vi "Create Mask.vi"(8 "Combine Masks? (F)":bool, 9 "1-Bit Mask Value (T)":bool=TRUE, 10 "Mask Color (Black)":u32(colorbox), 11 "image data":T1) -> (3 "image data":T1)   [LabVIEW 2017]
doc: "Applies a mask to an image and returns the mask information in the <B>mask</B> element of <B>image data</B>. This VI is useful if you want to make a certain color in an image transparent before writing the image to a 2D picture control."
uses:
  imagedata.ctl
panel:
  in  "Case Constant\n(See Context Help)":bool=TRUE
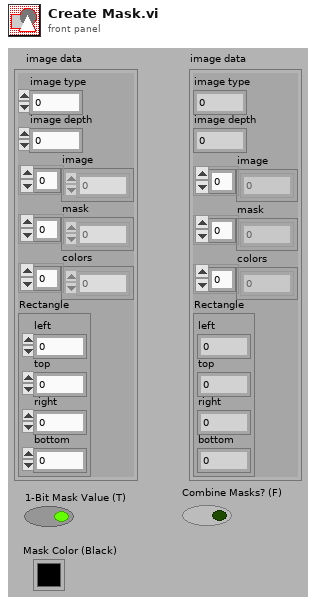
[diagram p1: front panel]
types:
  T1 = typedef "imagedata.ctl" = cluster{"image type":i32, "image depth":i32, "image":u8[], "mask":u8[], "colors":u32[], "Rectangle":cluster{"left":i16, "top":i16, "right":i16, "bottom":i16}}
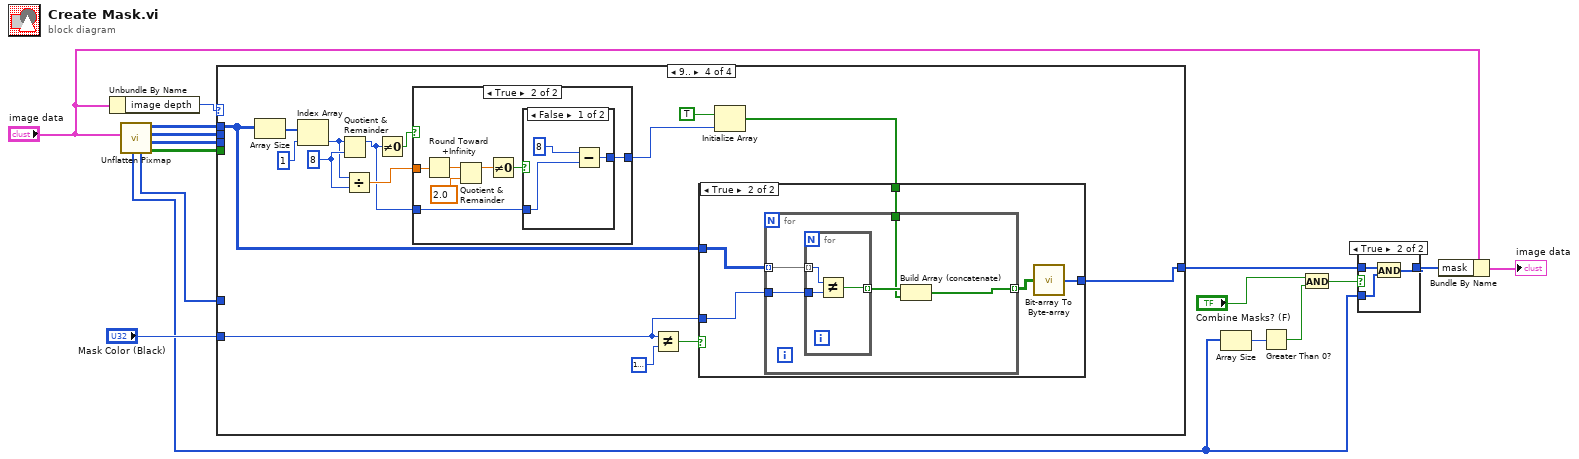
[diagram p0: block diagram]
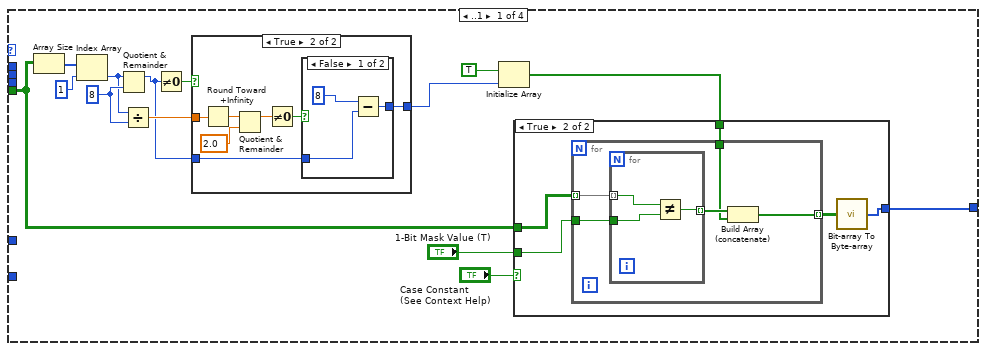
[diagram p3: hidden frame]
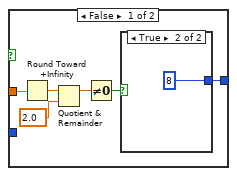
[diagram p4: hidden frame]
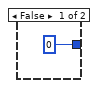
[diagram p5: hidden frame]
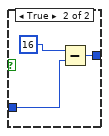
[diagram p6: hidden frame]
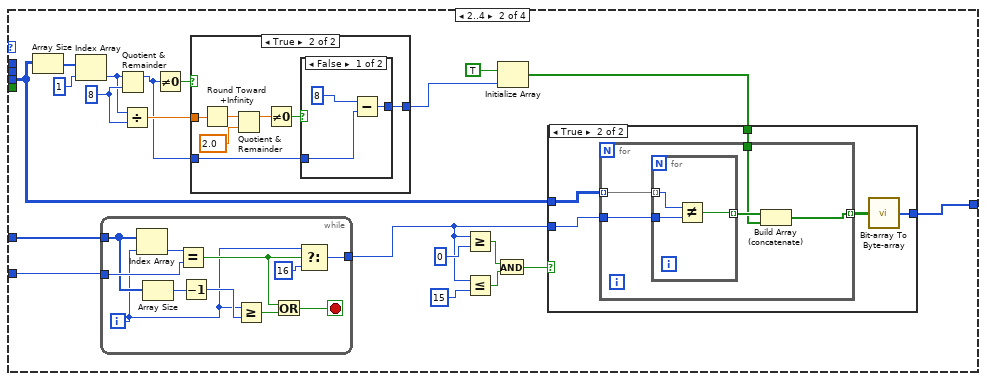
[diagram p8: hidden frame]
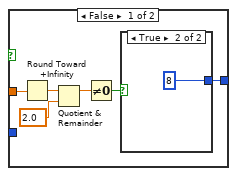
[diagram p9: hidden frame]
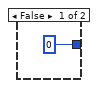
[diagram p10: hidden frame]
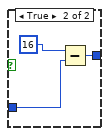
[diagram p11: hidden frame]
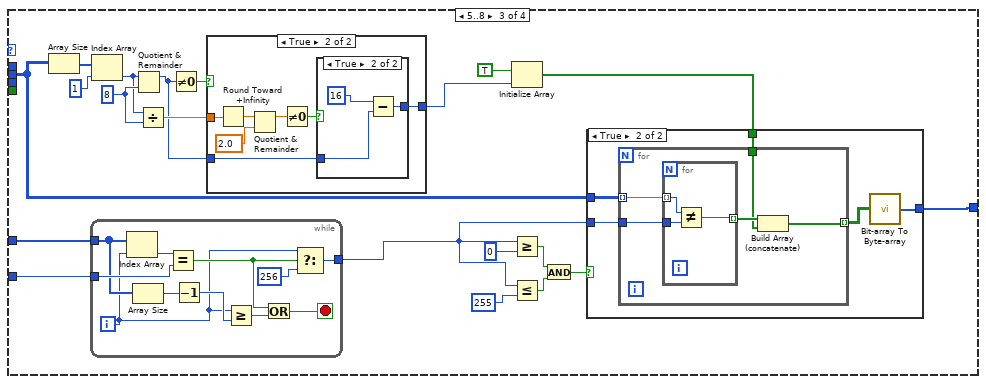
[diagram p13: hidden frame]
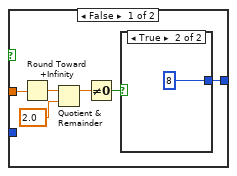
[diagram p14: hidden frame]
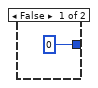
[diagram p15: hidden frame]
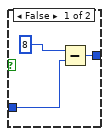
[diagram p16: hidden frame]
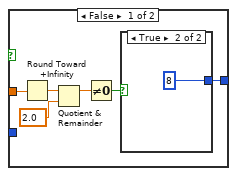
[diagram p18: hidden frame]
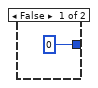
[diagram p19: hidden frame]
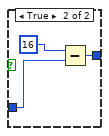
[diagram p20: hidden frame]
diagram:
  n1 = Unbundle By Name("image data") -> ("image depth"=w1:i32)
  n2 = call "Unflatten Pixmap.vi"("image data"="image data") -> ("1-bit pixmap"=w13:bool[][], "4-bit pixmap"=w14:u8[][], "8-bit pixmap"=w15:u8[][], "24-bit pixmap"=w16:u32[][], "colors"=w3:u32[], "mask"=w4:u8[])  [unwired: 4 in, 1 out]
  n3 = case shown="9.." w1 {
    tunnel: w15 -> [_ _ w140 _]
    tunnel: w14 -> [_ w77 _ _]
    tunnel: w13 -> [w24 _ _ _]
    tunnel: w16 -> [_ _ _ w198]
    tunnel: [w20 w71 w136 w200] -> w7
    tunnel: w3 -> [_ w70 w135 _]
    tunnel: "Mask Color (Black)" -> [_ w69 w134 w199]
    frame ..1 {
      w26 = 8 ("y")
      n4 = Array Size(array=w24) -> (size(s)=w28:i32[])
      n5 = Index Array(array=w28, index=1) -> (element=w22:i32)
      n6 = Quotient & Remainder(x=w22, y=w26) -> (x-y*floor(x/y)=w21:i32)  [unwired: 1 out]
      n7 = Divide(x=w22, y=w26) -> (x/y=w25:dbl)
      n8 = Not Equal To 0?(x=w21) -> (x != 0?=w27:bool)
      n9 = case shown="True" w27 {
        tunnel: w25 -> [w32 w45]
        tunnel: w21 -> [_ w40]
        tunnel: [w31 w39] -> w18
        frame False {
          n10 = Round Toward +Infinity(x=w32) -> (ceil(x): smallest int >= x=w33:dbl)
          n11 = Quotient & Remainder(x=w33, y=2.0) -> (x-y*floor(x/y)=w36:dbl)  [unwired: 1 out]
          n12 = Not Equal To 0?(x=w36) -> (x != 0?=w35:bool)
          n13 = case shown="True" w35 {
            tunnel: [0 8] -> w31
            frame False {
            }
            frame True {
            }
          }
        }
        frame True {
          n14 = Round Toward +Infinity(x=w45) -> (ceil(x): smallest int >= x=w44:dbl)
          n15 = Quotient & Remainder(x=w44, y=2.0) -> (x-y*floor(x/y)=w41:dbl)  [unwired: 1 out]
          n16 = Not Equal To 0?(x=w41) -> (x != 0?=w42:bool)
          n17 = case shown="False" w42 {
            tunnel: w40 -> [w46 w49]
            tunnel: [w47 w50] -> w39
            frame False {
              n18 = Subtract(x=8, y=w46) -> (x-y=w47:i32)
            }
            frame True {
              n19 = Subtract(x=16, y=w49) -> (x-y=w50:i32)
            }
          }
        }
      }
      n20 = Initialize Array(TRUE, w18) -> (w17:bool[])
      n21 = case shown="True" "Case Constant\n(See Context Help)" {
        tunnel: w24 -> [_ w56]
        tunnel: [_ w52] -> w20
        tunnel: "1-Bit Mask Value (T)" -> [_ w55]
        tunnel: w17 -> [_ w54]
        frame False {
        }
        frame True {
          n22 = for {
            tunnel: w56 -> [w61] mode=indexing
            tunnel: [w57] -> w53 mode=indexing
            tunnel: w55 -> [w60]
            tunnel: w54 -> [w58]
            n23 = for {
              tunnel: w61 -> [w62] mode=indexing
              tunnel: [w63] -> w59 mode=indexing
              tunnel: w60 -> [w64]
              n24 = Not Equal?(x=w62, y=w64) -> (x != y?=w63:bool)
            }
            n25 = Build Array (concatenate)(w59, w58) -> (w57:bool[])
          }
          n26 = call "Bit-array To Byte-array.vi"("bit array"=w53) -> ("byte array"=w52:u8[])
        }
      }
    }
    frame 2..4 {
      w79 = 8 ("y")
      n27 = Array Size(array=w77) -> (size(s)=w81:i32[])
      n28 = Index Array(array=w81, index=1) -> (element=w73:i32)
      n29 = while {
        tunnel: w70 -> [w93]
        tunnel: w69 -> [w94]
        tunnel: [w85] -> w68
        i -> [w87]
        stop <- w92 stop-if-true
        n30 = Index Array(array=w93, index=w87) -> (element=w95:u32)
        n31 = Array Size(array=w93) -> (size(s)=w90:i32)
        n32 = Equal?(x=w95, y=w94) -> (x = y?=w89:bool)
        n33 = Decrement(x=w90) -> (x-1=w88:i32)
        n34 = Greater Or Equal?(x=w87, y=w88) -> (x >= y?=w91:bool)
        n35 = Or(x=w89, y=w91) -> (x .or. y?=w92:bool)
        n36 = Select(t=w87, s=w89, f=16) -> (s? t:f=w85:i32)
      }
      n37 = Quotient & Remainder(x=w73, y=w79) -> (x-y*floor(x/y)=w72:i32)  [unwired: 1 out]
      n38 = Divide(x=w73, y=w79) -> (x/y=w78:dbl)
      n39 = Not Equal To 0?(x=w72) -> (x != 0?=w80:bool)
      n40 = case shown="True" w80 {
        tunnel: w78 -> [w97 w110]
        tunnel: w72 -> [_ w105]
        tunnel: [w96 w104] -> w66
        frame False {
          n41 = Round Toward +Infinity(x=w97) -> (ceil(x): smallest int >= x=w98:dbl)
          n42 = Quotient & Remainder(x=w98, y=2.0) -> (x-y*floor(x/y)=w101:dbl)  [unwired: 1 out]
          n43 = Not Equal To 0?(x=w101) -> (x != 0?=w100:bool)
          n44 = case shown="True" w100 {
            tunnel: [0 8] -> w96
            frame False {
            }
            frame True {
            }
          }
        }
        frame True {
          n45 = Round Toward +Infinity(x=w110) -> (ceil(x): smallest int >= x=w109:dbl)
          n46 = Quotient & Remainder(x=w109, y=2.0) -> (x-y*floor(x/y)=w106:dbl)  [unwired: 1 out]
          n47 = Not Equal To 0?(x=w106) -> (x != 0?=w107:bool)
          n48 = case shown="False" w107 {
            tunnel: w105 -> [w111 w114]
            tunnel: [w112 w115] -> w104
            frame False {
              n49 = Subtract(x=8, y=w111) -> (x-y=w112:i32)
            }
            frame True {
              n50 = Subtract(x=16, y=w114) -> (x-y=w115:i32)
            }
          }
        }
      }
      n51 = Greater Or Equal?(x=w68, y=u8 0) -> (x >= y?=w76:bool)
      n52 = Less Or Equal?(x=w68, y=u8 15) -> (x <= y?=w75:bool)
      n53 = And(x=w76, y=w75) -> (x .and. y?=w84:bool)
      n54 = Initialize Array(TRUE, w66) -> (w65:bool[])
      n55 = case shown="True" w84 {
        tunnel: w77 -> [_ w121]
        tunnel: w68 -> [_ w120]
        tunnel: w65 -> [_ w119]
        tunnel: [_ w117] -> w71
        frame False {
          (unwired) i16 0
          (unwired) i16 0
        }
        frame True {
          n56 = for {
            tunnel: w121 -> [w126] mode=indexing
            tunnel: [w122] -> w118 mode=indexing
            tunnel: w120 -> [w125]
            tunnel: w119 -> [w123]
            n57 = for {
              tunnel: w126 -> [w127] mode=indexing
              tunnel: [w128] -> w124 mode=indexing
              tunnel: w125 -> [w129]
              n58 = Not Equal?(x=w127, y=w129) -> (x != y?=w128:bool)
            }
            n59 = Build Array (concatenate)(w124, w123) -> (w122:bool[])
          }
          n60 = call "Bit-array To Byte-array.vi"("bit array"=w118) -> ("byte array"=w117:u8[])
        }
      }
    }
    frame 5..8 {
      w142 = 8 ("y")
      n61 = Array Size(array=w140) -> (size(s)=w144:i32[])
      n62 = while {
        tunnel: w135 -> [w158]
        tunnel: w134 -> [w159]
        tunnel: [w150] -> w133
        i -> [w152]
        stop <- w157 stop-if-true
        n63 = Index Array(array=w158, index=w152) -> (element=w160:u32)
        n64 = Array Size(array=w158) -> (size(s)=w155:i32)
        n65 = Equal?(x=w160, y=w159) -> (x = y?=w153:bool)
        n66 = Decrement(x=w155) -> (x-1=w154:i32)
        n67 = Greater Or Equal?(x=w152, y=w154) -> (x >= y?=w156:bool)
        n68 = Or(x=w153, y=w156) -> (x .or. y?=w157:bool)
        n69 = Select(t=w152, s=w153, f=256) -> (s? t:f=w150:i32)
      }
      n70 = Index Array(array=w144, index=1) -> (element=w138:i32)
      n71 = Quotient & Remainder(x=w138, y=w142) -> (x-y*floor(x/y)=w137:i32)  [unwired: 1 out]
      n72 = Divide(x=w138, y=w142) -> (x/y=w141:dbl)
      n73 = Not Equal To 0?(x=w137) -> (x != 0?=w143:bool)
      n74 = case shown="True" w143 {
        tunnel: w141 -> [w162 w175]
        tunnel: w137 -> [_ w170]
        tunnel: [w161 w169] -> w131
        frame False {
          n75 = Round Toward +Infinity(x=w162) -> (ceil(x): smallest int >= x=w163:dbl)
          n76 = Quotient & Remainder(x=w163, y=2.0) -> (x-y*floor(x/y)=w166:dbl)  [unwired: 1 out]
          n77 = Not Equal To 0?(x=w166) -> (x != 0?=w165:bool)
          n78 = case shown="True" w165 {
            tunnel: [0 8] -> w161
            frame False {
            }
            frame True {
            }
          }
        }
        frame True {
          n79 = Round Toward +Infinity(x=w175) -> (ceil(x): smallest int >= x=w174:dbl)
          n80 = Quotient & Remainder(x=w174, y=2.0) -> (x-y*floor(x/y)=w171:dbl)  [unwired: 1 out]
          n81 = Not Equal To 0?(x=w171) -> (x != 0?=w172:bool)
          n82 = case shown="True" w172 {
            tunnel: w170 -> [w176 w179]
            tunnel: [w177 w180] -> w169
            frame False {
              n83 = Subtract(x=8, y=w176) -> (x-y=w177:i32)
            }
            frame True {
              n84 = Subtract(x=16, y=w179) -> (x-y=w180:i32)
            }
          }
        }
      }
      n85 = Initialize Array(TRUE, w131) -> (w130:bool[])
      n86 = Greater Or Equal?(x=w133, y=u8 0) -> (x >= y?=w148:bool)
      n87 = Less Or Equal?(x=w133, y=u8 255) -> (x <= y?=w149:bool)
      n88 = And(x=w148, y=w149) -> (x .and. y?=w145:bool)
      n89 = case shown="True" w145 {
        tunnel: w140 -> [_ w186]
        tunnel: [_ w182] -> w136
        tunnel: w133 -> [_ w185]
        tunnel: w130 -> [_ w184]
        frame False {
        }
        frame True {
          n90 = for {
            tunnel: w186 -> [w191] mode=indexing
            tunnel: [w187] -> w183 mode=indexing
            tunnel: w185 -> [w190]
            tunnel: w184 -> [w188]
            n91 = for {
              tunnel: w191 -> [w194] mode=indexing
              tunnel: [w192] -> w189 mode=indexing
              tunnel: w190 -> [w193]
              n92 = Not Equal?(x=w194, y=w193) -> (x != y?=w192:bool)
            }
            n93 = Build Array (concatenate)(w189, w188) -> (w187:bool[])
          }
          n94 = call "Bit-array To Byte-array.vi"("bit array"=w183) -> ("byte array"=w182:u8[])
        }
      }
    }
    frame 9.. {
      w205 = 8 ("y")
      n95 = Array Size(array=w198) -> (size(s)=w207:i32[])
      n96 = Index Array(array=w207, index=1) -> (element=w203:i32)
      n97 = Quotient & Remainder(x=w203, y=w205) -> (x-y*floor(x/y)=w201:i32)  [unwired: 1 out]
      n98 = Divide(x=w203, y=w205) -> (x/y=w204:dbl)
      n99 = Not Equal To 0?(x=w201) -> (x != 0?=w206:bool)
      n100 = case shown="True" w206 {
        tunnel: w204 -> [w211 w224]
        tunnel: [w210 w219] -> w196
        tunnel: w201 -> [_ w218]
        frame False {
          n101 = Round Toward +Infinity(x=w211) -> (ceil(x): smallest int >= x=w212:dbl)
          n102 = Quotient & Remainder(x=w212, y=2.0) -> (x-y*floor(x/y)=w215:dbl)  [unwired: 1 out]
          n103 = Not Equal To 0?(x=w215) -> (x != 0?=w214:bool)
          n104 = case shown="True" w214 {
            tunnel: [0 8] -> w210
            frame False {
            }
            frame True {
            }
          }
        }
        frame True {
          n105 = Round Toward +Infinity(x=w224) -> (ceil(x): smallest int >= x=w223:dbl)
          n106 = Quotient & Remainder(x=w223, y=2.0) -> (x-y*floor(x/y)=w220:dbl)  [unwired: 1 out]
          n107 = Not Equal To 0?(x=w220) -> (x != 0?=w221:bool)
          n108 = case shown="False" w221 {
            tunnel: [w227 w230] -> w219
            tunnel: w218 -> [w226 w229]
            frame False {
              n109 = Subtract(x=8, y=w226) -> (x-y=w227:i32)
            }
            frame True {
              n110 = Subtract(x=16, y=w229) -> (x-y=w230:i32)
            }
          }
        }
      }
      n111 = Not Equal?(x=w199, y=u32 16777216) -> (x != y?=w209:bool)
      n112 = Initialize Array(TRUE, w196) -> (w195:bool[])
      n113 = case shown="True" w209 {
        tunnel: [_ w232] -> w200
        tunnel: w199 -> [_ w235]
        tunnel: w195 -> [_ w234]
        tunnel: w198 -> [_ w231]
        frame False {
        }
        frame True {
          n114 = for {
            tunnel: w231 -> [w239] mode=indexing
            tunnel: [w236] -> w233 mode=indexing
            tunnel: w235 -> [w240]
            tunnel: w234 -> [w237]
            n115 = for {
              tunnel: w239 -> [w243] mode=indexing
              tunnel: [w241] -> w238 mode=indexing
              tunnel: w240 -> [w242]
              n116 = Not Equal?(x=w243, y=w242) -> (x != y?=w241:bool)
            }
            n117 = Build Array (concatenate)(w238, w237) -> (w236:bool[])
          }
          n118 = call "Bit-array To Byte-array.vi"("bit array"=w233) -> ("byte array"=w232:u8[])
        }
      }
    }
  }
  n119 = Array Size(array=w4) -> (size(s)=w10:i32)
  n120 = Greater Than 0?(x=w10) -> (x > 0?=w8:bool)
  n121 = And(x="Combine Masks? (F)", y=w8) -> (x .and. y?=w9:bool)
  n122 = case shown="True" w9 {
    tunnel: w7 -> [w244 w247]
    tunnel: [w244 w245] -> w11
    tunnel: w4 -> [_ w246]
    frame False {
    }
    frame True {
      n123 = And(x=w247, y=w246) -> (x .and. y?=w245:u8[])
    }
  }
  n124 = Bundle By Name(cluster="image data", "mask"=w11) -> (→"image data":T1)
